vi "Tosca-Start AI Recording.vi"(0 "Path":path, 11 "error in (no error)":errorcluster) -> (15 "error out":errorcluster)   [LabVIEW 2020]
uses:
  epl-vi-lib/TCP VIs/TCP Params.ctl
  3a7128ec-ff33-4f91-882c-7a4c4875f354.vi
  epl-vi-lib/TCP VIs/TCP Write.vi
  Tosca-Globals.vi
  epl-vi-lib/Utility VIs/File IO VIs/Read Write Anything/Read Anything.vi
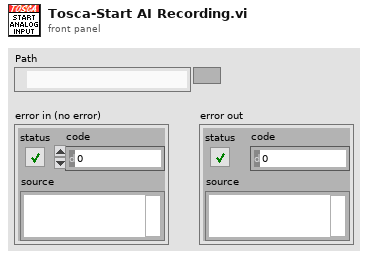
[diagram p1: front panel]
types:
  T1 = enum16{"big-endian, network order", "native, host order", "little-endian"}
  T2 = typedef "TCP Params.ctl" = cluster{"IP Address":string, "Port":i32}
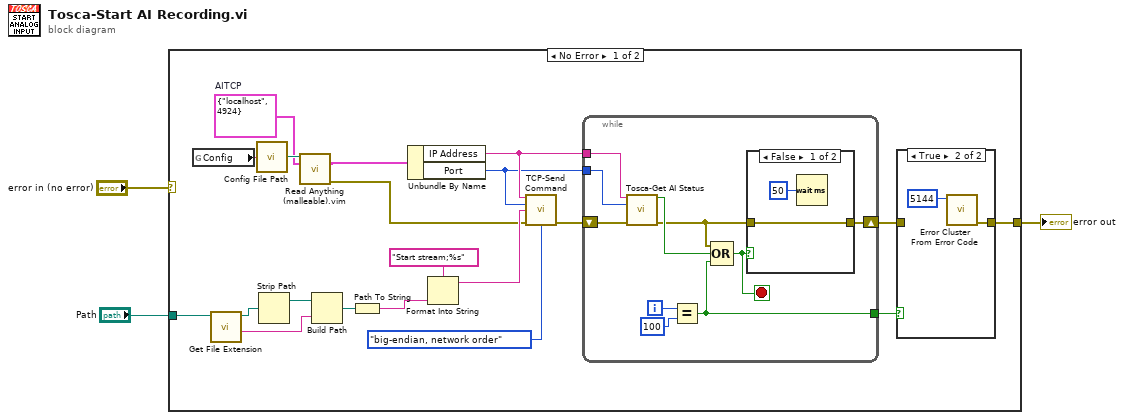
[diagram p0: block diagram]
diagram:
  n1 = case shown="No Error" "error in (no error)" {
    selector: "error in (no error)" -> [_ w40]
    tunnel: [w17 w40] -> w2
    tunnel: "Path" -> [w23 _]
    frame No Error {
      w7 = T2 {"IP Address"="localhost", "Port"=4924}  # AITCP
      n2 = global read "Tosca-Globals.vi" "Config"() -> (w9:string)
      n3 = call <vilib>:"Get File Extension.vi"("file"=w23) -> ("filename without extension"=w12:string, "dup file"=w21:path)  [unwired: 6 in, 3 out]
      n4 = call "Config File Path.vi"("AppName"=w9) -> ("Default config file name"=w8:path)
      n5 = Strip Path(path=w21) -> (stripped path=w13:path)  [unwired: 1 out]
      n6 = call "Read Anything (malleable).vim"("Config file path"=w8, "Options in"=w7) -> ("Options out"=w6:T2, "error out"=w5:errorcluster)  [unwired: 10 in, 2 out]
      n7 = Build Path(base path=w13, name or relative path=w12) -> (appended path=w11:path)
      n8 = Path To String(path=w11) -> (string=w10:string)
      n9 = Unbundle By Name(w6) -> ("IP Address"=w20:string, "Port"=w19:i32)
      n10 = Format Into String(format string="Start stream;%s", w10) -> (resulting string=w14:string)  [unwired: 2 in, 1 out]
      n11 = call "TCP-Send Command.vi"("PXI Address"=w20, "Port"=w19, "Command"=w14, "error in (no error)"=w5, "byte order"=T1."big-endian, network order") -> ("error out"=w18:errorcluster)  [unwired: 10 in]
      n12 = while {
        tunnel: w20 -> [w33]
        tunnel: w19 -> [w32]
        shift-right: [w28] -> w15
        shift-left: w18 -> [w31]
        tunnel: [w25] -> w16
        i -> [w27]
        stop <- w26 stop-if-true
        n13 = call "Tosca-Get AI Status.vi"("IP Address"=w33, "Port"=w32, "error in (no error)"=w31) -> ("Recording"=w30:bool, "error out"=w29:errorcluster)  [unwired: 11 in]
        n14 = Equal?(x=w27, y=100) -> (x = y?=w25:bool)
        n15 = Compound Arithmetic op=OR(w29, w30, w25) -> (w26:bool)
        n16 = case shown="False" w26 {
          tunnel: w29 -> [w34 w36]
          tunnel: [w34 w36] -> w28
          frame False {
            n17 = Wait (ms)(milliseconds to wait=u32 50) -> ()  [unwired: 1 out]
          }
          frame True {
          }
        }
      }
      n18 = case shown="True" w16 {
        tunnel: w15 -> [w37 _]
        tunnel: [w37 w39] -> w17
        frame False {
        }
        frame True {
          n19 = call <vilib>:"Error Cluster From Error Code.vi"("error code (0)"=5144) -> ("error out"=w39:errorcluster)  [unwired: 8 in]
        }
      }
    }
    frame Error {
    }
  }
  "error out" <- w2
